vi "AutoUpdate.vi"() -> (0 "error out":errorcluster caption="错误输出", 3 "return code":i32 caption="返回代码")   [LabVIEW 2011]
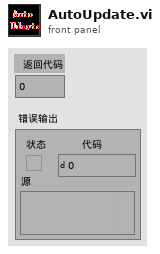
[diagram p1: front panel]
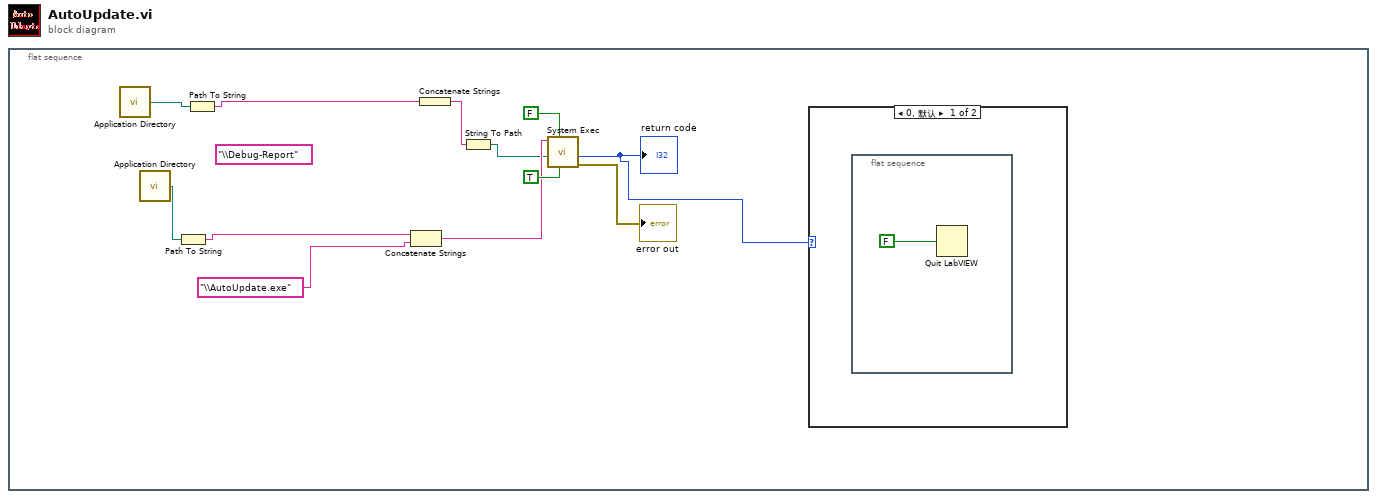
[diagram p0: block diagram]
diagram:
  n1 = flat-sequence {
    frame #0 {
      (unwired) "\\Debug-Report" ("字符串")
      n2 = call <vilib>:"Application Directory.vi"() -> ("Application Directory"=w10:path)
      n3 = call <vilib>:"Application Directory.vi"() -> ("Application Directory"=w12:path)
      n4 = Path To String(path=w12) -> (string=w11:string)
      n5 = Path To String(path=w10) -> (string=w9:string)
      n6 = Concatenate Strings(w11, "\\AutoUpdate.exe" ("字符串")) -> (w2:string)
      n7 = Concatenate Strings(w9) -> (w8:string)
      n8 = String To Path(string=w8) -> (path=w1:path)
      n9 = call <vilib>:"System Exec.vi"("run minimized? (F)"=TRUE, "wait until completion? (T)"=FALSE, "working directory"=w1, "command line"=w2) -> ("error out"=→"error out":errorcluster, "return code"=w5:i32)  [unwired: 4 in, 2 out]
      "return code" <- w5
      n10 = case shown="0, 默认" w5 {
        frame 0, Default {
          n11 = flat-sequence {
            frame #0 {
              n12 = Quit LabVIEW(quit? (T)=FALSE ("退出？(T)")) -> ()
            }
          }
        }
        frame 1 {
        }
      }
    }
  }
